vi "Ventana-Padre_Hijo-SubVI.vi"(1 "error in (no error)":errorcluster, 2 "Child Window Name":string, 3 "Parent Window Name":string) -> (0 "error out":errorcluster)   [LabVIEW 2018]
uses:
  user32.dll
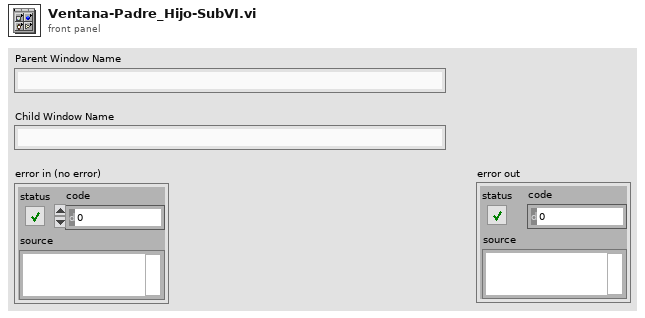
[diagram p1: front panel]
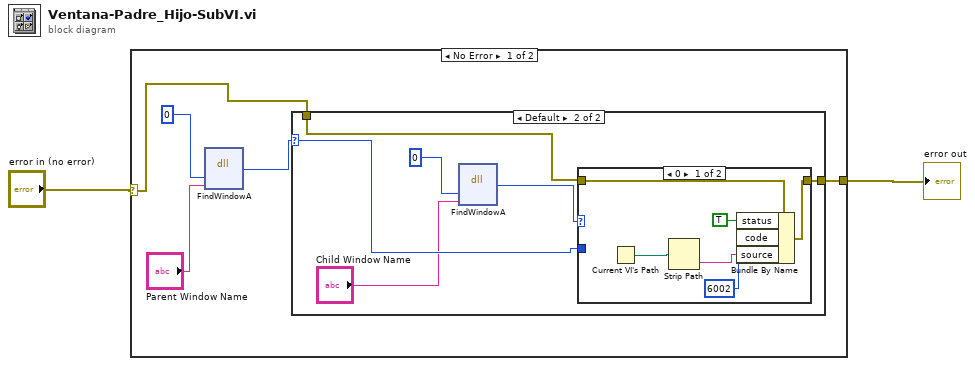
[diagram p0: block diagram]
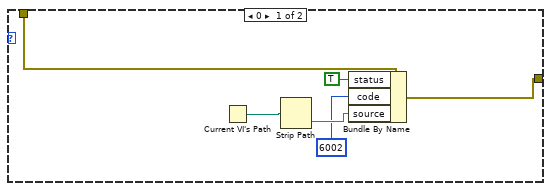
[diagram p2: hidden frame]
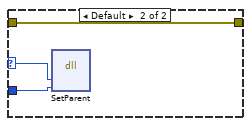
[diagram p3: hidden frame]
diagram:
  n1 = case shown="No Error" "error in (no error)" {
    selector: "error in (no error)" -> [w4 w29]
    tunnel: [w3 w29] -> w1
    frame No Error {
      n2 = dll-call lib="user32.dll" fn="FindWindowA" label="FindWindow"("IpszClassName"=0, "IpszWindowName"="Parent Window Name") -> ("hWnd"=w6:u32)  [unwired: 5 in, 2 out]
      n3 = case shown="Default" w6 {
        selector: w6 -> [_ w18]
        tunnel: w4 -> [w8 w15]
        tunnel: [w9 w14] -> w3
        frame 0 {
          n4 = Current VI's Path() -> (path=w12:path)
          n5 = Strip Path(path=w12) -> (name=w13:string)  [unwired: 1 out]
          n6 = Bundle By Name(cluster=w8, "status"=TRUE, "code"=6002, "source"=w13) -> (w9:errorcluster)
        }
        frame Default {
          n7 = dll-call lib="user32.dll" fn="FindWindowA" label="FindWindow"("IpszClassName"=0, "IpszWindowName"="Child Window Name") -> ("hWnd"=w19:u32)  [unwired: 5 in, 2 out]
          n8 = case shown="0" w19 {
            selector: w19 -> [_ w28]
            tunnel: w18 -> [_ w27]
            tunnel: w15 -> [w24 w26]
            tunnel: [w20 w26] -> w14
            frame 0 {
              n9 = Current VI's Path() -> (path=w25:path)
              n10 = Strip Path(path=w25) -> (name=w21:string)  [unwired: 1 out]
              n11 = Bundle By Name(cluster=w24, "status"=TRUE, "code"=6002, "source"=w21) -> (w20:errorcluster)
            }
            frame Default {
              n12 = dll-call lib="user32.dll" fn="SetParent" label="Set Parent"("Child"=w28, "NewParent"=w27) -> ()  [unwired: 6 in, 2 out]
            }
          }
        }
      }
    }
    frame Error {
    }
  }
  "error out" <- w1
